vi "VisionBasedAlignment.vi"() -> ()   [LabVIEW 2016]
panel:
  in  "Theta":dbl format="%#_13g"
  in  "Z":dbl format="%#_13g"
  in  "X":dbl format="%#_13g"
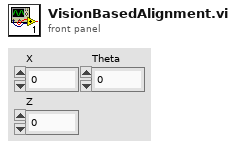
[diagram p1: front panel]
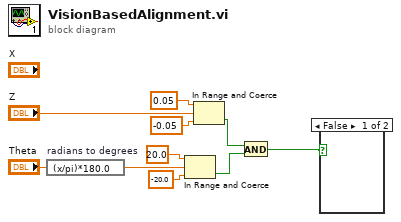
[diagram p0: block diagram]
diagram:
  n1 = expression code="(x/pi)*180.0" "radians to degrees"("Theta") -> (w8:dbl)
  n2 = In Range and Coerce(upper limit=20.0, x=w8, lower limit=-20.0) -> (In Range?=w6:bool)  [unwired: 1 out]
  n3 = In Range and Coerce(upper limit=0.05, x="Z", lower limit=-0.05) -> (In Range?=w4:bool)  [unwired: 1 out]
  n4 = And(x=w4, y=w6) -> (x .and. y?=w1:bool)
  n5 = case shown="False" w1 {
    frame False {
    }
    frame True {
    }
  }
